vi "Overwrite-all-variables.vi"(8 "error in (no error)":errorcluster, 10 "Temp. vars.":T1 {"Temperature characteristics"."Stand. dev. temperature" format="%#.1f"; "Temperature characteristics"."Min. temperature" format="%#.0f"; "Temperature characteristics"."Max. temperature" format="%#.0f"; "Temperature characteristics"."Average temperature" format="%#.0f"}, 11 "Temp. params. ref. in":refnum<data-value>) -> (0 "error out":errorcluster, 3 "Temp. params. ref.":refnum<data-value>)   [LabVIEW 2013, in "CameraVision.lvlib" / "CV-Temperature.lvclass"]
uses:
  CV-Temperature.lvclass
  Temperature-variables.ctl
  Temperature-characteristics.ctl
  UI/Module-states.ctl
  CV-Temperature.lvclass/CV-Temperature.ctl
  UI/CV-UI.lvclass
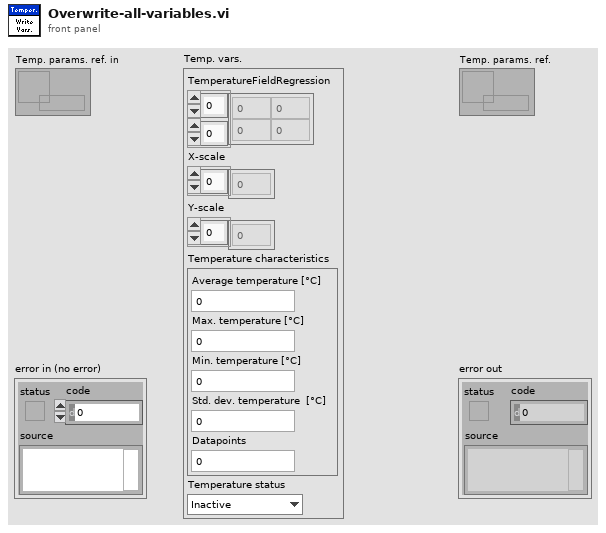
[diagram p1: front panel]
types:
  T1 = typedef "CameraVision.lvlib/CV-Temperature.lvclass/Temperature-variables.ctl" = cluster{"TemperatureFieldRegression":dbl[][], "X-scale":sgl[], "Y-scale":sgl[], "Temperature characteristics":T2, "Temperature status":T3}
  T2 = typedef "CameraVision.lvlib/CV-Temperature.lvclass/Temperature-characteristics.ctl" = cluster{"Average temperature ":dbl, "Max. temperature":dbl, "Min. temperature":dbl, "Stand. dev. temperature":dbl, "Datapoints":dbl}
  T3 = typedef "CameraVision.lvlib/CV-UI.lvclass/Module-states.ctl" = enum16{"Inactive", "Active", "Data-loss", "Error", "Simulation", "Synchronizing", "Initialized", "Released"}
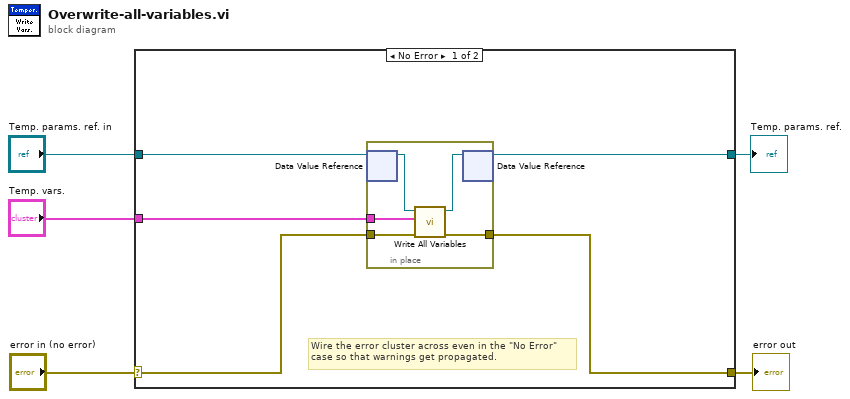
[diagram p0: block diagram]
diagram:
  n1 = case shown="No Error" "error in (no error)" {
    selector: "error in (no error)" -> [w8 w17]
    tunnel: [w9 w17] -> w4
    tunnel: "Temp. params. ref. in" -> [w7 w16]
    tunnel: "Temp. vars." -> [w10 _]
    tunnel: [w6 w16] -> w1
    frame No Error {
      # "Wire the error cluster across even in the \"No Error\"\ncase so that warnings get propagated."
      n2 = in-place {
        in-place-border: w10 -> [w15]
        in-place-border: [w14] -> w9
        in-place-border: w8 -> [w13]
        n3 = in-place-dvr #1(w7) -> (w12:refnum<class "CV-Temperature.lvclass">)  [unwired: 1 out]
        n4 = call "Write All Variables.vi"("error in (no error)"=w13, "Temp. vars."=w15, "Temp params in"=w12) -> ("error out"=w14:errorcluster, "Temp params out"=w11:refnum<class "CV-Temperature.lvclass">)  [unwired: 7 in]
        n5 = in-place-dvr #1(w11) -> (w6:refnum<data-value>)  [unwired: 1 out]
      }
    }
    frame Error {
    }
  }
  "error out" <- w4
  "Temp. params. ref." <- w1
